vi "JSON to MultiD Array.vi"(8 "error in (no error)":errorcluster, 9 "ArrayElementType":variant, 10 "NDims":i32, 11 "JSON Value in":refnum<class "JSON Value.lvclass">) -> (0 "error out":errorcluster, 2 "Dimensions":i32[](array[numeric]), 3 "Array Elements":variant[](array[variant]))   [LabVIEW 2011, in "Variant JSON.lvlib"]
uses:
  Variant JSON.lvlib
  JSON Value/JSON Value.lvclass
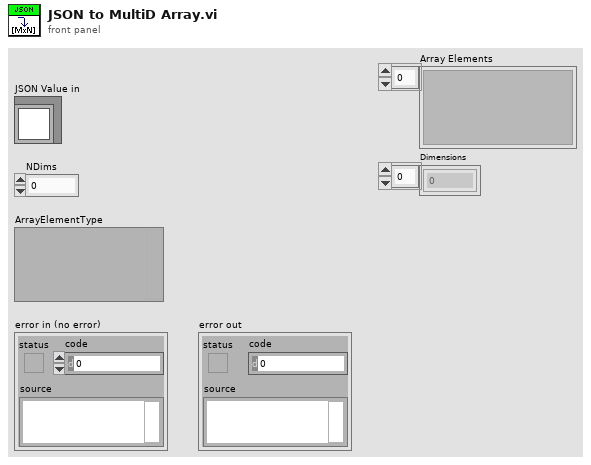
[diagram p1: front panel]
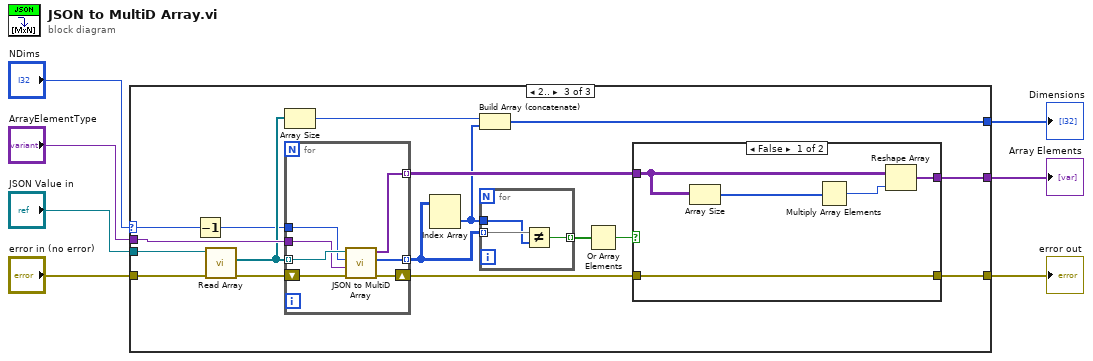
[diagram p0: block diagram]
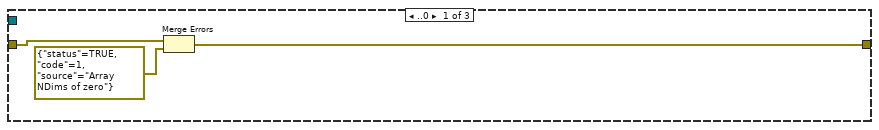
[diagram p2: hidden frame]
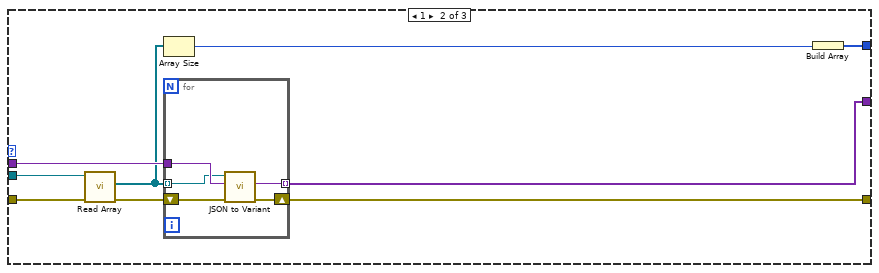
[diagram p3: hidden frame]
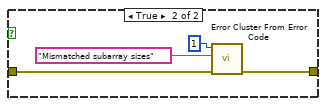
[diagram p4: hidden frame]
diagram:
  n1 = case shown="2.." "NDims" {
    selector: "NDims" -> [_ _ w37]
    tunnel: [w9 w15 w29] -> w3
    tunnel: "JSON Value in" -> [_ w19 w41]
    tunnel: "ArrayElementType" -> [_ w18 w40]
    tunnel: "error in (no error)" -> [w10 w17 w39]
    tunnel: [_ w14 w35] -> w2
    tunnel: [_ w11 w27] -> w1
    frame ..0 {
      n2 = Merge Errors(w10, errorcluster {"status"=TRUE, "code"=1, "source"="Array NDims of zero"} ("error in")) -> (w9:errorcluster)
    }
    frame 1 {
      n3 = call-dynamic "Read Array.vi"("error in (no error)"=w17, "JSON Value In"=w19) -> ("error out"=w16:errorcluster, "Array"=w13:refnum<class "JSON Value.lvclass">[])  [unwired: 7 in, 1 out]
      n4 = Array Size(array=w13) -> (size(s)=w12:i32)
      n5 = for {
        tunnel: w18 -> [w24]
        shift-right: [w22] -> w15
        shift-left: w16 -> [w23]
        tunnel: w13 -> [w21] mode=indexing
        tunnel: [w20] -> w14 mode=indexing
        n6 = call "JSON to Variant.vi"("error in (no error)"=w23, "Variant (Data Type)"=w24, "JSON Value"=w21) -> ("error out"=w22:errorcluster, "Variant out"=w20:variant)  [unwired: 7 in]
      }
      n7 = Build Array(w12) -> (w11:i32[])
    }
    frame 2.. {
      n8 = Decrement(x=w37) -> (x-1=w25:i32)
      n9 = call-dynamic "Read Array.vi"("error in (no error)"=w39, "JSON Value In"=w41) -> ("error out"=w38:errorcluster, "Array"=w34:refnum<class "JSON Value.lvclass">[])  [unwired: 7 in, 1 out]
      n10 = Array Size(array=w34) -> (size(s)=w33:i32)
      n11 = for {
        tunnel: w40 -> [w58]
        shift-right: [w56] -> w28
        shift-left: w38 -> [w57]
        tunnel: w34 -> [w60] mode=indexing
        tunnel: w25 -> [w59]
        tunnel: [w55] -> w36 mode=indexing
        tunnel: [w54] -> w32 mode=indexing
        n12 = call "JSON to MultiD Array.vi"("error in (no error)"=w57, "ArrayElementType"=w58, "NDims"=w59, "JSON Value in"=w60) -> ("error out"=w56:errorcluster, "Dimensions"=w54:i32[], "Array Elements"=w55:variant[])  [unwired: 5 in]
      }
      n13 = Index Array(array=w32) -> (element=w26:i32[])  [unwired: 2 in]
      n14 = Build Array (concatenate)(w33, w26) -> (w27:i32[])
      n15 = for {
        tunnel: w32 -> [w44] mode=indexing
        tunnel: [w43] -> w31 mode=indexing
        tunnel: w26 -> [w42]
        n16 = Not Equal?(x=w44, y=w42) -> (x != y?=w43:bool)
      }
      n17 = Or Array Elements(Boolean array=w31) -> (logical OR=w30:bool)
      n18 = case shown="False" w30 {
        tunnel: w36 -> [w47 _]
        tunnel: [w46 _] -> w35
        tunnel: [w45 w53] -> w29
        tunnel: w28 -> [w45 w52]
        frame False {
          n19 = Array Size(array=w47) -> (size(s)=w48:i32[])
          n20 = Multiply Array Elements(1:w48) -> (0:w49:i32)
          n21 = Reshape Array(w47, w49) -> (w46:variant[])
        }
        frame True {
          n22 = call <vilib>:"Error Cluster From Error Code.vi"("error in (no error)"=w52, "error message (\"\")"="Mismatched subarray sizes" ("error message (\"\")"), "error code (0)"=1) -> ("error out"=w53:errorcluster)  [unwired: 6 in]
        }
      }
    }
  }
  "error out" <- w3
  "Array Elements" <- w2
  "Dimensions" <- w1
